vi "Test_URI_Class.vi"(8 "error in (no error)":errorcluster) -> (0 "error out":errorcluster)   [LabVIEW 2013]
uses:
  source/uri/URI.lvclass/URI.ctl
  source/components/path/URI-Component.Path.lvclass/URI-Component.Path.ctl
  source/components/query/URI-Component.Query.lvclass/URI-Component.Query.ctl
  source/uri/Read scheme.vi
  source/uri/Read username.vi
  source/uri/Read password.vi
  source/uri/Read host.vi
  source/uri/Read port.vi
  source/uri/Read path.vi
  source/uri/Read path segments.vi
  source/uri/Read Query.vi
  source/uri/Read fragment.vi
  source/utilities/Percent-Encode String.vi
  source/components/path/Get Segments.vi
  source/components/query/Get Key-Value Pairs.vi
  source/utilities/isHEXDigit.vi
  <vilib>/addons/_JKI Toolkits/Caraya/classes/Assert/Assert Equal Value_Variant.vi
  <vilib>/addons/_JKI Toolkits/Caraya/classes/Assert/Assert Equal Value and Type_Variant.vi
  source/components/path/Get path (absolute).vi
  <vilib>/Utility/error.llb/Trim Whitespace.vi
  <vilib>/addons/_JKI Toolkits/Caraya/classes/Test/Test.lvclass
  <vilib>/addons/_JKI Toolkits/Caraya/classes/Assert/Assert.lvclass
  source/uri/URI.lvclass
  source/openURI.lvlib
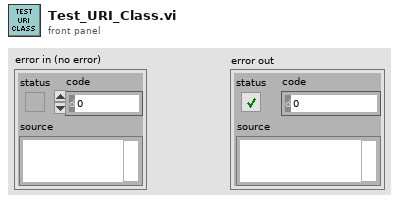
[diagram p1: front panel]
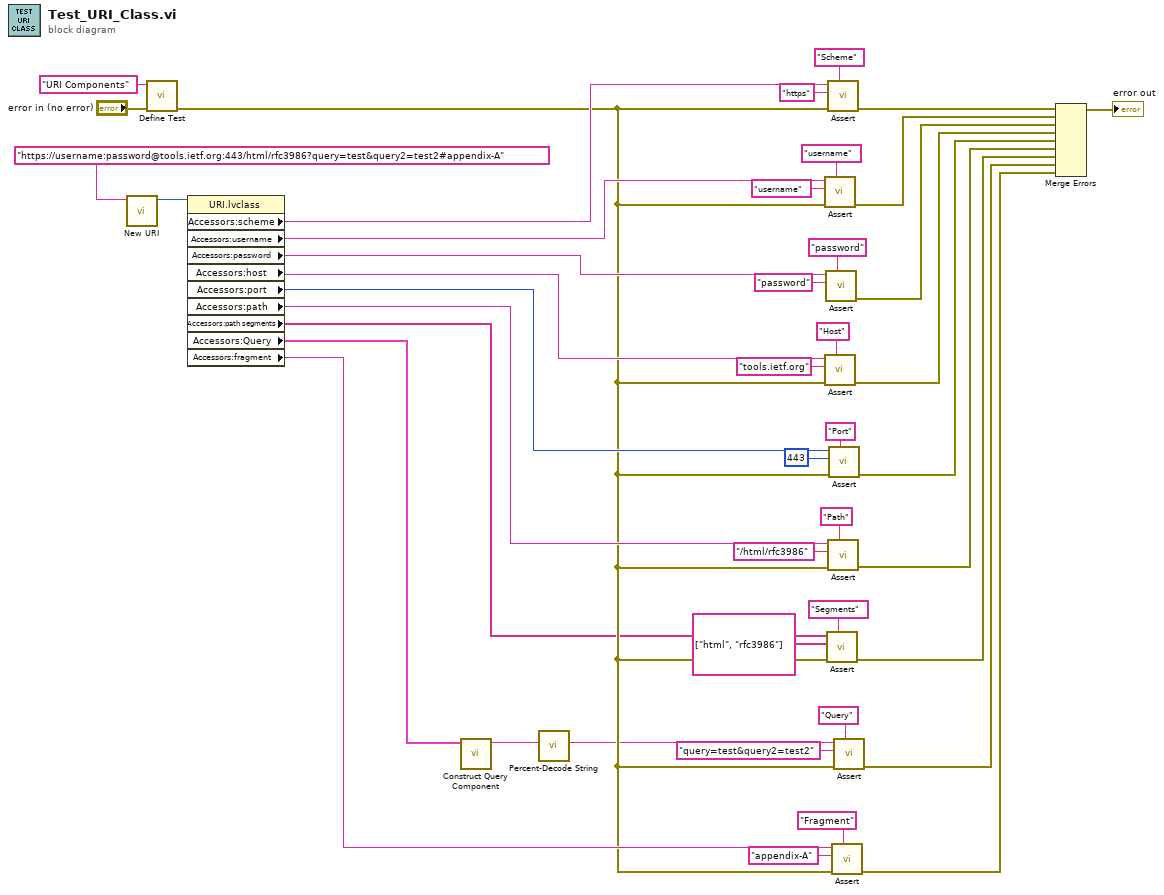
[diagram p0: block diagram]
diagram:
  n1 = call "New URI.vi"("URI"="https://username:password@tools.ietf.org:443/html/rfc3986?query=test&query2=test2#appendix-A") -> ("URI"=w39:refnum<class "URI.lvclass">)  [unwired: 9 in, 1 out]
  n2 = call <vilib>:"Define Test.vi"("error in (no error)"="error in (no error)", "Label (VI Title)"="URI Components") -> ("error out"=w5:errorcluster)  [unwired: 9 in]
  n3 = property on="Property Node" class="URI.lvclass"(reference=w39) -> ("Accessors:scheme"=w38:string, "Accessors:username"=w29:string, "Accessors:password"=w24:string, "Accessors:host"=w34:string, "Accessors:port"=w22:u16, "Accessors:path"=w16:string, "Accessors:path segments"=w1:string[], "Accessors:Query"=w8:cluster{"argument":string, "value":string}[], "Accessors:fragment"=w10:string)  [unwired: 1 in, 2 out]
  n4 = call "Construct Query Component.vi"("Query"=w8) -> ("query"=w3:string)  [unwired: 10 in]
  n5 = call "Percent-Decode String.vi"("Pct-Encoded String"=w3) -> ("String"=w2:string)  [unwired: 10 in]
  n6 = call-poly <vilib>:"Assert.vi"("Label"="username" ("URI"), "error in (no error)"=w5, "Y"="username" ("URI"), "X"=w29) -> ("error out"=w28:errorcluster)  [unwired: 7 in]
  n7 = call-poly <vilib>:"Assert.vi"("Label"="Host" ("URI"), "error in (no error)"=w5, "Y"="tools.ietf.org" ("URI"), "X"=w34) -> ("error out"=w32:errorcluster)  [unwired: 7 in]
  n8 = call-poly <vilib>:"Assert.vi"("Label"="password" ("URI"), "Y"="password" ("URI"), "X"=w24) -> ("error out"=w25:errorcluster)  [unwired: 8 in]
  n9 = call-poly <vilib>:"Assert.vi"("Label"="Segments" ("URI"), "error in (no error)"=w5, "Y"=string[] ["html", "rfc3986"] ("Segments"), "X"=w1) -> ("error out"=w13:errorcluster)  [unwired: 7 in]
  n10 = call-poly <vilib>:"Assert.vi"("Label"="Scheme" ("URI"), "error in (no error)"=w5, "Y"="https" ("URI"), "X"=w38) -> ("error out"=w33:errorcluster)  [unwired: 7 in]
  n11 = call-poly <vilib>:"Assert.vi"("Label"="Path" ("URI"), "error in (no error)"=w5, "Y"="/html/rfc3986" ("URI"), "X"=w16) -> ("error out"=w17:errorcluster)  [unwired: 7 in]
  n12 = call-poly <vilib>:"Assert.vi"("Label"="Port" ("URI"), "error in (no error)"=w5, "Y"=u16 443 ("port"), "X"=w22) -> ("error out"=w20:errorcluster)  [unwired: 7 in]
  n13 = call-poly <vilib>:"Assert.vi"("Label"="Fragment" ("URI"), "error in (no error)"=w5, "Y"="appendix-A" ("URI"), "X"=w10) -> ("error out"=w9:errorcluster)  [unwired: 7 in]
  n14 = call-poly <vilib>:"Assert.vi"("Label"="Query" ("URI"), "error in (no error)"=w5, "Y"="query=test&query2=test2" ("URI"), "X"=w2) -> ("error out"=w4:errorcluster)  [unwired: 7 in]
  n15 = Merge Errors(w33, w28, w25, w32, w20, w17, w13, w4, w9) -> (→"error out":errorcluster)
